vi "Single SSC DCPower Fill Additional Error info.vi"(0 "DCPower SSC in":T1, 11 "error in":errorcluster, 12 "previous error in":errorcluster) -> (15 "error out":errorcluster)   [LabVIEW 2019]
doc: "This VI appends information to the error message from the SSC cluster if an error is on error in, but not initial error.\n\nThis makes it easier to debug code since you know what session/site/channel/pin actually threw the error."
uses:
  SSC DCPower.ctl
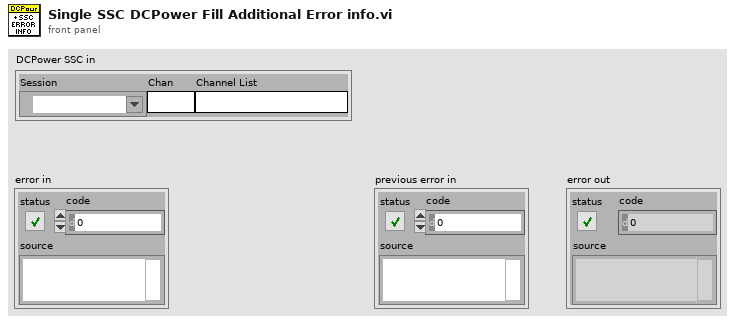
[diagram p1: front panel]
types:
  T1 = typedef "SSC DCPower.ctl" = cluster{"Session":refnum<k15>, "Chan":string, "Channel List":string}
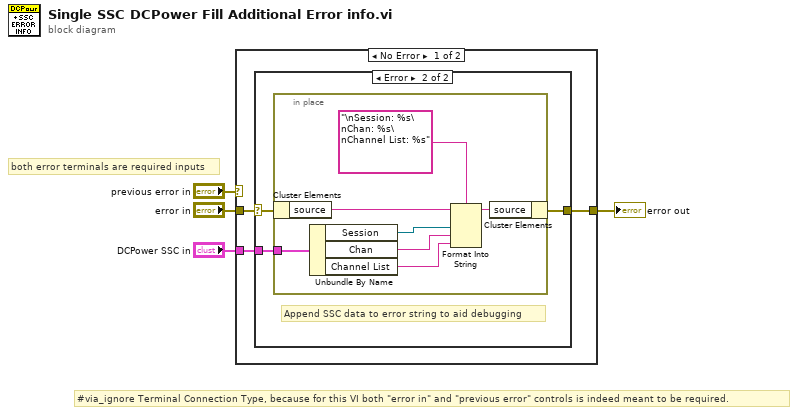
[diagram p0: block diagram]
diagram:
  # "#via_ignore Terminal Connection Type, because for this VI both \"error in\" and \"previous error\" controls is indeed meant to be required."
  # "both error terminals are required inputs"
  n1 = case shown="No Error" "previous error in" {
    selector: "previous error in" -> [_ w19]
    tunnel: [w6 w19] -> w3
    tunnel: "error in" -> [w7 _]
    tunnel: "DCPower SSC in" -> [w5 _]
    frame No Error {
      n2 = case shown="Error" w7 {
        selector: w7 -> [w8 w11]
        tunnel: [w8 w9] -> w6
        tunnel: w5 -> [_ w10]
        frame No Error {
        }
        frame Error {
          # "Append SSC data to error string to aid debugging"
          n3 = in-place {
            in-place-border: w10 -> [w16]
            n4 = in-place-cluster #1(w11) -> ("source"=w18:string)
            n5 = Unbundle By Name(w16) -> ("Session"=w15:refnum<k15>, "Chan"=w14:string, "Channel List"=w13:string)
            n6 = Format Into String(format string="\nSession: %s\nChan: %s\nChannel List: %s", initial string=w18, w15, w14, w13) -> (resulting string=w17:string)  [unwired: 1 in, 1 out]
            n7 = in-place-cluster #1("source"=w17) -> (w9:errorcluster)
          }
        }
      }
    }
    frame Error {
      # "These errors already existed, leave them as they are"
    }
  }
  "error out" <- w3
